vi "DateChecker.vi"() -> ()   [LabVIEW 2024]
uses:
  <vilib>/Utility/error.llb/Trim Whitespace One-Sided.vi
  CV_Shared_Library/CV_Shared_Library.lvlib
  <userlib>/_OpenG.lib/string/string.llb/openg_string.lvlib
panel:
  in  "omit list path":path=path "D:/Comics/data/dl_manager/Date Check Omit List.txt"
  out "current vol":string
  in  "stop":bool
  out "Array":string[](array[string])
  out "error out":errorcluster
  in  "cv issues":path=path "D:/Comics/data/cv_issues"
  in  "cv vols":path=path "D:/Comics/data/cv_volumes"
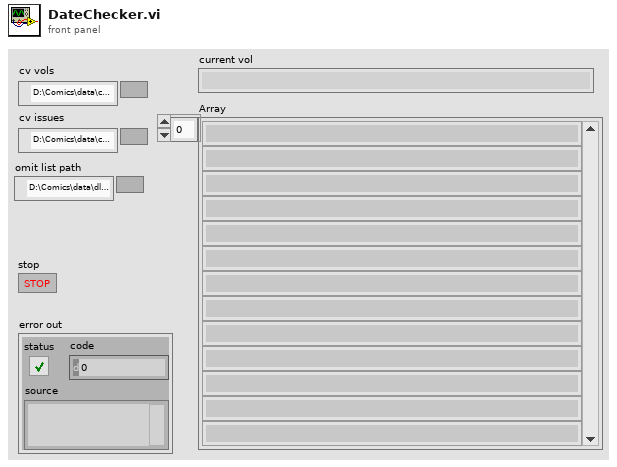
[diagram p1: front panel]
types:
  T1 = typedef "CV_RESTful_Lib.lvlib/local_volume--cluster.ctl" = cluster{"id":i32, "name":string, "sortable_name":string, "aliases":string[], "description":string, "site_detail_url":string, "count_of_issues":i32, "start_year":i32, "publisher_id":i32, "issue_ids":i32[], "date_last_updated":timestamp, "volume":i32, "cv_id":string, "volume type":T2}
  T2 = typedef "CV_Shared_Library.lvlib/volume.type--enum.ctl" = enum16{"Ongoing", "Limited Series", "Annual", "One Shot", "Reprint/Document", "Star Comics", "Epic Comics"}
  T3 = typedef "CV_RESTful_Lib.lvlib/local_issue--cluster.ctl" = cluster{"cover_date":timestamp, "id":i32, "cv_id":string, "name":string, "sortable_name":string, "issue_number":string, "deck":string, "description":string, "volume":T4, "store_date":timestamp, "date_last_updated":timestamp, "site_detail_url":string, "cover_url":string, "associated_images":T5[], "characters":T4[], "concepts":T4[], "creators":T6[], "storyArcs":T4[], "teams":T4[], "in collection":bool}
  T4 = typedef "CV_RESTful_Lib.lvlib/cv_issue.generic_credit--cluster.ctl" = cluster{"id":i32, "name":string}
  T5 = typedef "CV_RESTful_Lib.lvlib/cv_issue.associated_image--cluster.ctl" = cluster{"original_url":string, "id":i32}
  T6 = typedef "CV_RESTful_Lib.lvlib/cv_issue.person_credit--cluster.ctl" = cluster{"id":i32, "name":string, "role":string}
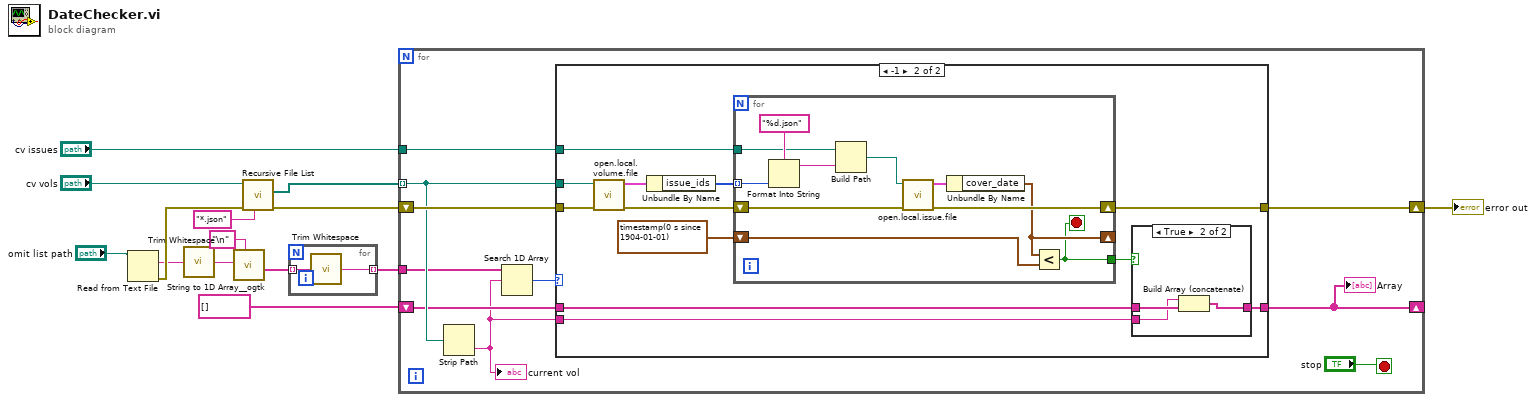
[diagram p0: block diagram]
diagram:
  n1 = Read from Text File(file (use dialog)="omit list path") -> (text=w5:string, error out=w7:errorcluster)  [unwired: 3 in, 2 out]
  n2 = call <vilib>:"Trim Whitespace.vi"("string"=w5) -> ("trimmed string"=w4:string)  [unwired: 1 in]
  n3 = call <userlib>:"String to 1D Array__ogtk.vi"("delimiter (Tab)"="\n", "string"=w4) -> ("Array of Strings"=w2:string[])  [unwired: 9 in]
  n4 = call <vilib>:"Recursive File List.vi"("pattern"="*.json", "error in (no error)"=w7, "Folder Path"="cv vols") -> ("error out"=w12:errorcluster, "All Files in Dir"=w11:path[])  [unwired: 4 in, 3 out]
  n5 = for {
    tunnel: w2 -> [w16] mode=indexing
    tunnel: [w15] -> w1 mode=indexing
    n6 = call <vilib>:"Trim Whitespace.vi"("string"=w16) -> ("trimmed string"=w15:string)  [unwired: 1 in]
  }
  n7 = for {
    tunnel: w11 -> [w23] mode=indexing
    shift-right: [w24] -> w9
    shift-left: w12 -> [w26]
    tunnel: "cv issues" -> [w25]
    shift-right: [w20] -> _
    shift-left: string[] [] -> [w21]
    tunnel: w1 -> [w19]
    stop <- "stop" stop-if-true
    n8 = Strip Path(path=w23) -> (name=w18:string)  [unwired: 1 out]
    "current vol" <- w18
    n9 = Search 1D Array(1D array=w19, element=w18) -> (index of element=w17:i32)  [unwired: 1 in]
    n10 = case shown="-1" w17 {
      tunnel: w26 -> [w28 w40]
      tunnel: w25 -> [_ w37]
      tunnel: [w28 w35] -> w24
      tunnel: w23 -> [_ w33]
      tunnel: w21 -> [w27 w31]
      tunnel: [w27 w30] -> w20
      tunnel: w18 -> [_ w29]
      frame Default {
      }
      frame -1 {
        n11 = call "open.local.volume.file.vi"("error in (no error)"=w40, "volume json"=w33) -> ("error out"=w36:errorcluster, "volume"=w39:T1)  [unwired: 8 in]
        n12 = Unbundle By Name(w39) -> ("issue_ids"=w38:i32[])
        n13 = for {
          tunnel: w38 -> [w54] mode=indexing
          tunnel: w37 -> [w52]
          shift-right: [w50] -> w35
          shift-left: w36 -> [w51]
          shift-right: [w47] -> _
          shift-left: timestamp(0 s since 1904-01-01) -> [w46]
          tunnel: [w45] -> w32
          stop <- w45 stop-if-true
          n14 = Format Into String(format string="%d.json", w54) -> (resulting string=w53:string)  [unwired: 2 in, 1 out]
          n15 = Build Path(base path=w52, name or relative path=w53) -> (appended path=w49:path)
          n16 = call "open.local.issue.file.vi"("error in (no error)"=w51, "issue json path"=w49) -> ("error out"=w50:errorcluster, "issue"=w48:T3)  [unwired: 8 in]
          n17 = Unbundle By Name(w48) -> ("cover_date"=w47:timestamp)
          n18 = Less?(x=w47, y=w46) -> (x < y?=w45:bool)
        }
        n19 = case shown="True" w32 {
          tunnel: w31 -> [w41 w44]
          tunnel: [w41 w43] -> w30
          tunnel: w29 -> [_ w42]
          frame False {
          }
          frame True {
            n20 = Build Array (concatenate)(w42, w44) -> (w43:string[])
          }
        }
      }
    }
    "Array" <- w20
  }
  "error out" <- w9
